vi "LibXML_FreeXPath.vi"(8 "error in":errorcluster, 11 "XPathObj":u32) -> (0 "error out":errorcluster)   [LabVIEW 2019, in "Tools.lvlib" / "LibXML.lvlib"]
doc: "Release the Pointer to the XPath Obj. This should be used for all XPathObjs."
uses:
  LibXML.lvlib
  dll/libxml2.dll
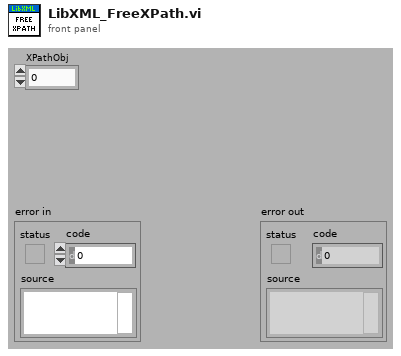
[diagram p1: front panel]
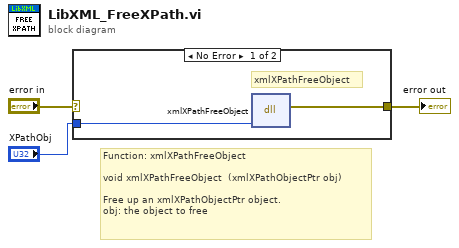
[diagram p0: block diagram]
diagram:
  # "Function: xmlXPathFreeObject\n\nvoid\txmlXPathFreeObject\t\t(xmlXPathObjectPtr obj)\n\nFree up an xmlXPathObjectPtr object.\nobj:\tthe object to free"
  n1 = case shown="No Error" "error in" {
    selector: "error in" -> [_ w6]
    tunnel: [w4 w6] -> w2
    tunnel: "XPathObj" -> [w5 _]
    frame No Error {
      # "xmlXPathFreeObject"
      n2 = dll-call lib="C:/Projects/_Prywatne/MyCIT/Framework/Tools/XML/LibXML/dll/libxml2.dll" fn="xmlXPathFreeObject"("XPathObj"=w5) -> (error out=w4:errorcluster)  [unwired: 5 in, 1 out]
    }
    frame Error {
    }
  }
  "error out" <- w2
